vi "Testing01.vi"() -> ()   [LabVIEW 2012]
uses:
  Logging VIs/Controls/LoggingDevRef.ctl
  Logging VIs/Update VIs/Logging Update - Numeric.vi
  femtoRoboLib.lvlib
panel:
  out "LoggingDevRef":T1
  in  "Set":bool
  in  "Tree":string(tree)
  in  "Reload":bool
  in  "Value":dbl
  in  "Name":string
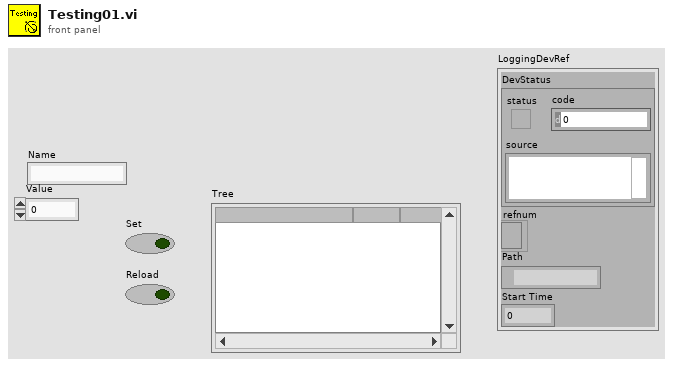
[diagram p1: front panel]
types:
  T1 = typedef "femtoRoboLib.lvlib/LoggingDevRef.ctl" = cluster{"DevStatus":errorcluster, "refnum":refnum<file>, "Path":path, "Start Time":u32}
  T2 = typedef "femtoRoboLib.lvlib/Log Entry - Full Block.ctl" = cluster{"Entries":T3[], "Time":u32}
  T3 = typedef "femtoRoboLib.lvlib/Log Entry.ctl" = cluster{"Name":string, "Type":T4, "Value":T5}
  T4 = typedef "femtoRoboLib.lvlib/Log Value Type.ctl" = enum16{"Boolean", "Numeric", "String", "Boolean Array", "Numeric Array", "String Array"}
  T5 = typedef "femtoRoboLib.lvlib/Log Value Cluster.ctl" = cluster{"Boolean Array":bool[], "Boolean":bool, "Numeric Array":dbl[], "Numeric":dbl, "String Array":string[], "String":string}
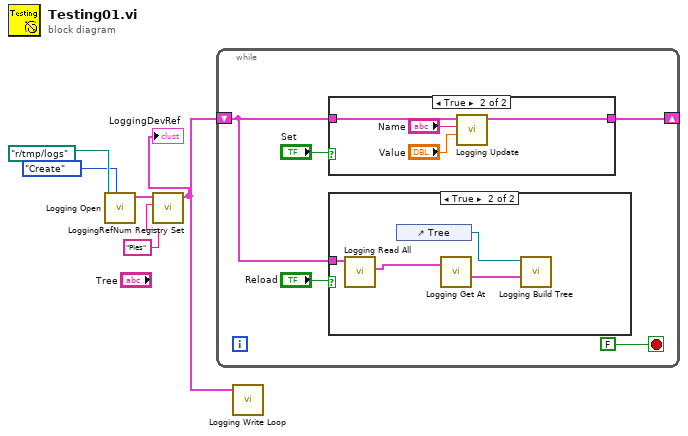
[diagram p0: block diagram]
diagram:
  n1 = call "Logging Open.vi"("Mode"=enum16{"Create", "Open"}."Create", "base path"=path "r:/tmp/logs" ("palette path")) -> ("LoggingDevRef"=w3:T1)  [unwired: 7 in, 1 out]
  n2 = call "LoggingRefNum Registry Set.vi"("refnum name"="Pies", "LoggingDevRef"=w3) -> ("LoggingDevRef"=w2:T1)  [unwired: 8 in, 1 out]
  "LoggingDevRef" <- w2
  n3 = while {
    shift-right: [w6] -> _
    shift-left: w2 -> [w10]
    stop <- FALSE stop-if-true
    n4 = case shown="True" "Set" {
      tunnel: w10 -> [w11 w15]
      tunnel: [w11 w12] -> w6
      frame False {
      }
      frame True {
        n5 = call-poly "Logging Update.vi"("Value"="Value", "Name"="Name", "LoggingDevRef"=w15) -> ("LoggingDevRef"=w12:T1)  [unwired: 3 in, 1 out]
      }
    }
    n6 = case shown="True" "Reload" {
      tunnel: w10 -> [_ w18]
      frame False {
      }
      frame True {
        n7 = call "Logging Read All.vi"("LoggingDevRef"=w18) -> ("Log"=w17:T2[])  [unwired: 4 in, 2 out]
        n8 = control-ref of="Tree"() -> (w16:refnum<vi>)
        n9 = call "Logging Get At.vi"("Log Input"=w17) -> ("Output"=w19:T2)  [unwired: 1 in]
        n10 = call "Logging Build Tree.vi"("Entries"=w19, "TreeRef"=w16) -> ()  [unwired: 5 in, 1 out]
      }
    }
  }
  n11 = call "Logging Write Loop.vi"("LoggingDevRef"=w2) -> ()  [unwired: 5 in]
